vi "Headers (Write).vi"(8 "error in (no error)":errorcluster, 10 "Headers":refnum<class "Headers.lvclass">, 11 "obj in":refnum<class "RequestBuilder.lvclass">) -> (0 "error out":errorcluster, 2 "success":bool, 3 "obj out":refnum<class "RequestBuilder.lvclass">)   [LabVIEW 2020, in "reqwest.lvlib" / "RequestBuilder.lvclass"]
uses:
  RequestBuilder.lvclass
  RequestBuilder.lvclass/RequestBuilder.ctl
  Headers/Headers.lvclass
  lv_reqwest_64.dll
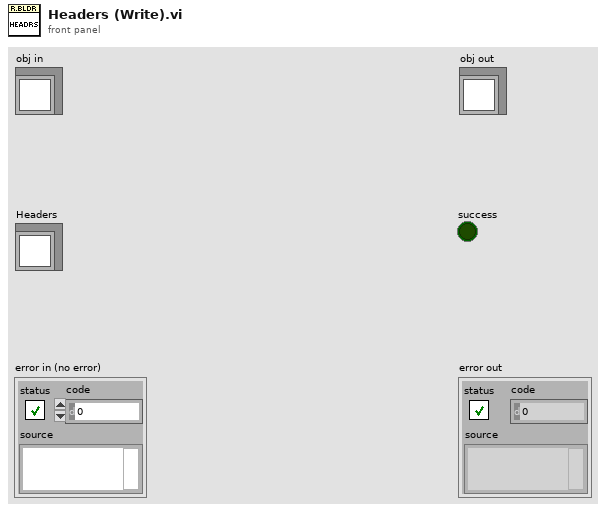
[diagram p1: front panel]
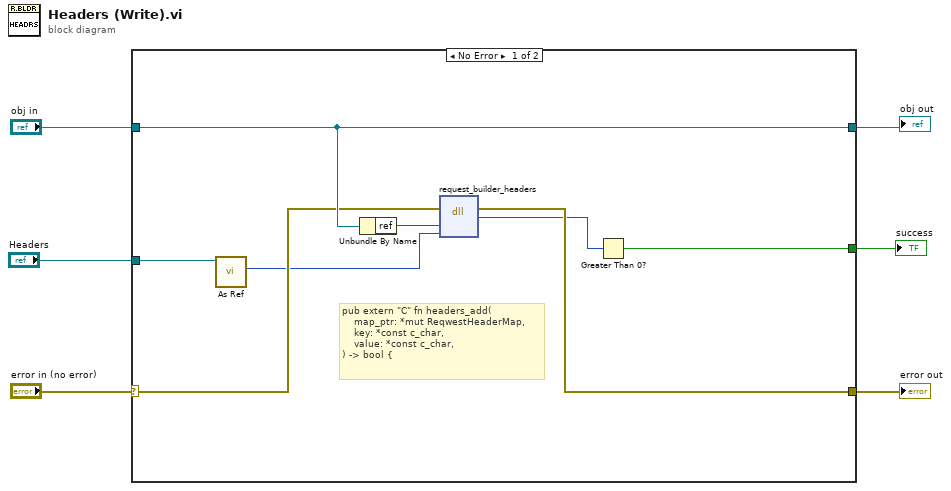
[diagram p0: block diagram]
diagram:
  n1 = case shown="No Error" "error in (no error)" {
    selector: "error in (no error)" -> [w13 w15]
    tunnel: "obj in" -> [w14 w16]
    tunnel: [w12 w15] -> w3
    tunnel: [w14 w16] -> w4
    tunnel: [w9 _] -> w2
    tunnel: "Headers" -> [w8 _]
    frame No Error {
      # "pub extern \"C\" fn headers_add(\n    map_ptr: *mut ReqwestHeaderMap,\n    key: *const c_char,\n    value: *const c_char,\n) -> bool {"
      n2 = call "As Ref.vi"("Headers in"=w8) -> ("ref"=w7:u64)  [unwired: 10 in]
      n3 = Unbundle By Name(w14) -> ("ref"=w11:u64)
      n4 = dll-call lib="C:/Projects/reqwest-rs-labview/lv_src/lv_reqwest_*.*" fn="request_builder_headers"(error in=w13, "request_builder_ref"=w11, "header_ref"=w7) -> (error out=w12:errorcluster, "result"=w10:u8)  [unwired: 4 in, 1 out]
      n5 = Greater Than 0?(x=w10) -> (x > 0?=w9:bool)
    }
    frame Error {
    }
  }
  "error out" <- w3
  "obj out" <- w4
  "success" <- w2
